vi "THD.vi"(0 "spectra":T2(array[cluster]), 9 "system info in":refnum<class "EP System Info.lvclass">, 11 "error in (no error)":errorcluster) -> (4 "THD [%]":dbl[](array[numeric]), 10 "system info out":refnum<class "EP System Info.lvclass">, 15 "error out":errorcluster)   [LabVIEW 2014, in "NI_EP_Power Quality.lvlib"]
doc: "Calculates the total harmonic distortion (THD) of voltage spectra, harmonic spectra, or spectra that contain both voltage and current as defined in IEC 61000-4-7:2009. This VI calculates the THD for all harmonics up to the 40th order as defined in EN 50160:2007.\n\nThis VI supports measuring single-line and multiple-line systems."
uses:
  <vilib>/addons/Electrical Power/PQ/NI_EP_Power Quality.lvlib
  <vilib>/addons/Electrical Power/PQ/Common/Controls/ep_AI Data Channel.ctl
  <vilib>/addons/Electrical Power/PQ/Common/Classes/System Info/EP System Info.lvclass
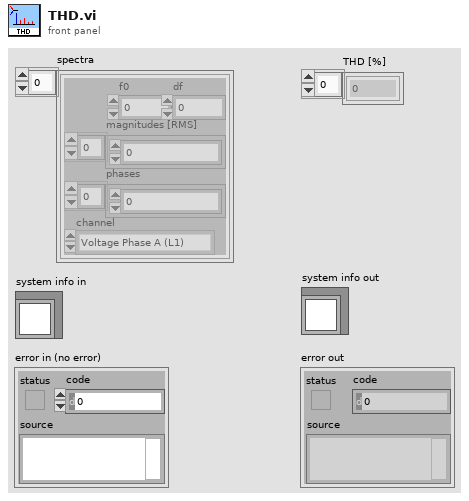
[diagram p1: front panel]
types:
  T1 = typedef "NI_EP_Power Quality.lvlib/ep_AI Data Channel.ctl" = enum16{"Voltage Phase A (L1)", "Voltage Phase B (L2)", "Voltage Phase C (L3)", "Voltage Phase N (Neutral)", "Current Phase A (L1)", "Current Phase B (L2)", "Current Phase C (L3)", "Current Phase N (Neutral)"}
  T2 = cluster{"f0":dbl, "df":dbl, "magnitudes [RMS]":dbl[], "phases":dbl[], "channel":T1}[]
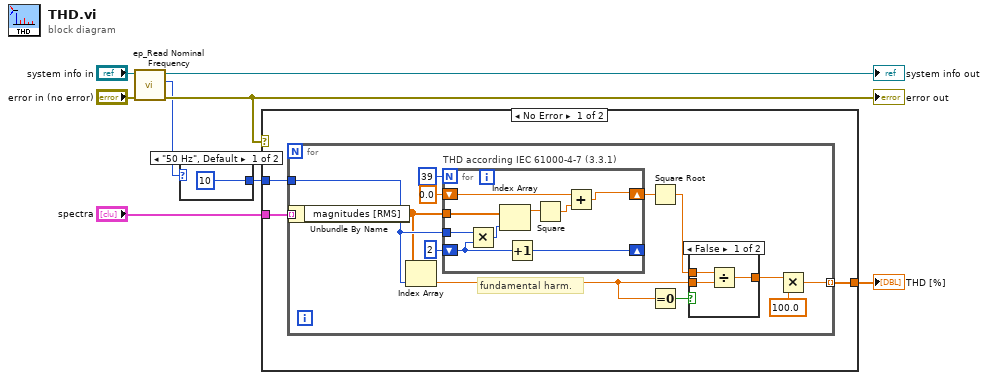
[diagram p0: block diagram]
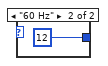
[diagram p2: hidden frame]
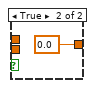
[diagram p3: hidden frame]
diagram:
  n1 = call <vilib>:"ep_Read Nominal Frequency.vi"("error in (no error)"="error in (no error)", "system info in"="system info in") -> ("error out"=w3:errorcluster, "nominal frequency"=w2:enum16{"50 Hz", "60 Hz"}, "system info out"=→"system info out":refnum<class "EP System Info.lvclass">)  [unwired: 6 in, 1 out]
  "error out" <- w3
  n2 = case shown="\"50 Hz\", Default" w2 {
    tunnel: [10 ("index") 12 ("index")] -> w1
    frame "50 Hz", Default {
    }
    frame "60 Hz" {
    }
  }
  n3 = case shown="No Error" w3 {
    tunnel: "spectra" -> [w13 _]
    tunnel: w1 -> [w12 _]
    tunnel: [w11 _] -> w5
    frame No Error {
      n4 = for {
        tunnel: w13 -> [w26] mode=indexing
        tunnel: w12 -> [w16]
        tunnel: [w15] -> w11 mode=indexing
        # "fundamental harm."
        n5 = Unbundle By Name(w26) -> ("magnitudes [RMS]"=w14:dbl[])
        n6 = Index Array(array=w14, index=w16) -> (element=w25:dbl)
        n7 = for "THD according IEC 61000-4-7 (3.3.1)" {
          N: 39 -> [_]
          shift-right: [w33] -> w20
          shift-left: 0.0 -> [w34]
          tunnel: w16 -> [w38]
          tunnel: w14 -> [w37]
          shift-right: [w32] -> _
          shift-left: 2 -> [w31]
          n8 = Multiply(x=w38, y=w31) -> (x*y=w39:i32)
          n9 = Index Array(array=w37, index=w39) -> (element=w36:dbl)
          n10 = Increment(x=w31) -> (x+1=w32:i32)
          n11 = Square(x=w36) -> (x^2=w35:dbl)
          n12 = Add(x=w34, y=w35) -> (x+y=w33:dbl)
        }
        n13 = Square Root(x=w20) -> (sqrt(x)=w23:dbl)
        n14 = Equal To 0?(x=w25) -> (x = 0?=w21:bool)
        n15 = case shown="False" w21 {
          tunnel: w25 -> [w28 _]
          tunnel: [w27 0.0 ("t")] -> w24
          tunnel: w23 -> [w29 _]
          frame False {
            n16 = Divide(x=w29, y=w28) -> (x/y=w27:dbl)
          }
          frame True {
          }
        }
        n17 = Multiply(x=w24, y=100.0) -> (x*y=w15:dbl)
      }
    }
    frame Error {
    }
  }
  "THD [%]" <- w5
